vi "unset metadata property.vi"(8 "error in":errorcluster, 10 "key":string, 11 "configuration in":refnum<class "TBM configuration.lvclass">) -> (0 "error out":errorcluster, 3 "configuration out":refnum<class "TBM configuration.lvclass">)   [LabVIEW 2013, in "TBM configuration.lvclass"]
doc: "Clears a key/value pair stored in the configuration object."
uses:
  TBM configuration.lvclass
  TBM configuration.lvclass/TBM configuration.ctl
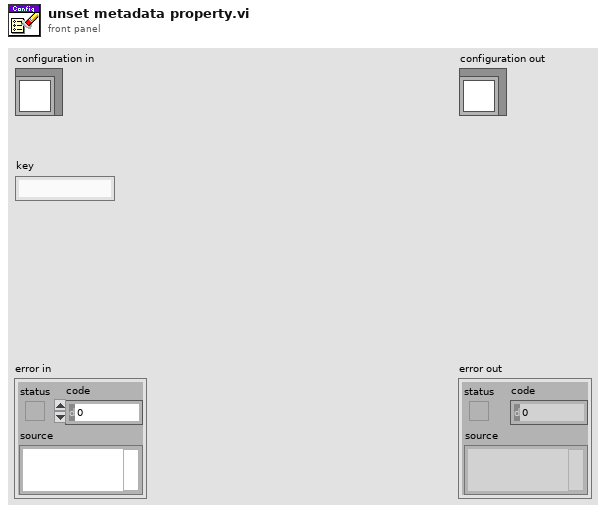
[diagram p1: front panel]
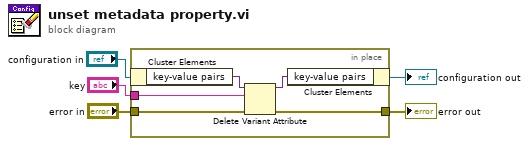
[diagram p0: block diagram]
diagram:
  n1 = in-place {
    in-place-border: "key" -> [w7]
    in-place-border: "error in" -> [w6]
    in-place-border: [w10] -> w1
    n2 = in-place-cluster #1("configuration in") -> ("key-value pairs"=w8:variant)
    n3 = Delete Variant Attribute(4:w6, 6:w7, 7:w8) -> (0:w10:errorcluster, 3:w9:variant)  [unwired: 1 out]
    n4 = in-place-cluster #1("key-value pairs"=w9) -> (→"configuration out":refnum<class "TBM configuration.lvclass">)
  }
  "error out" <- w1
